vi "Close Instrument Safely.vi"(8 "error in (no error)":errorcluster, 10 "Running (F)":bool, 11 "VISA Refnum in":refnum<visa-resource-name>) -> (0 "error out":errorcluster)   [LabVIEW 2020, in "Mock Temperature Controller.lvlib" / "Instrument Manager.lvlib"]
doc: "Stops the pump if it is running, clears the character buffer on the pump, and closes the VISA resources given."
uses:
  process loops/Instrument Manager/Instrument Manager.lvlib
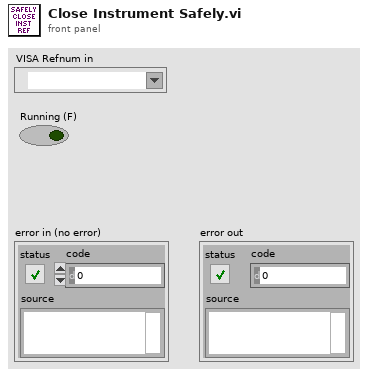
[diagram p1: front panel]
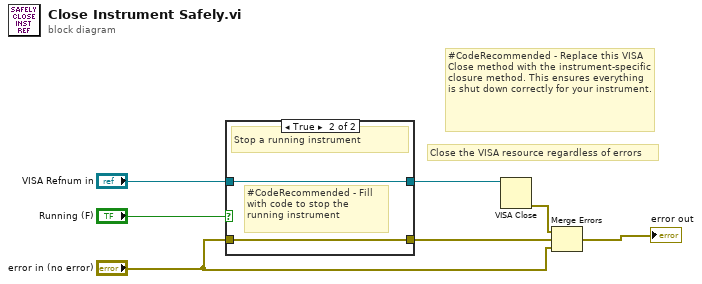
[diagram p0: block diagram]
diagram:
  # "#CodeRecommended - Replace this VISA Close method with the instrument-specific closure method. This ensures everything is shut down correctly for your instrument."
  # "Close the VISA resource regardless of errors"
  n1 = case shown="True" "Running (F)" {
    tunnel: "error in (no error)" -> [w9 w10]
    tunnel: [w9 w10] -> w2
    tunnel: "VISA Refnum in" -> [w8 w11]
    tunnel: [w8 w11] -> w5
    frame False {
    }
    frame True {
      # "#CodeRecommended - Fill with code to stop the\nrunning instrument"
      # "Stop a running instrument"
    }
  }
  n2 = VISA Close(VISA resource name=w5) -> (error out=w1:errorcluster)  [unwired: 1 in]
  n3 = Merge Errors(w1, w2, "error in (no error)") -> (→"error out":errorcluster)
